vi "Get Incrementing Class Name.vi"() -> (3 "String":string)   [LabVIEW 2020, in "New Class Dialog.lvclass"]
uses:
  New Class Dialog.lvclass
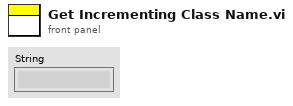
[diagram p1: front panel]
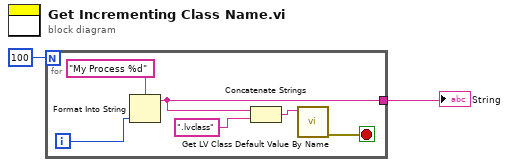
[diagram p0: block diagram]
diagram:
  n1 = for {
    N: 100 -> [_]
    tunnel: [w5] -> w2
    i -> [w7]
    stop <- w6 stop-if-true
    n2 = Format Into String(format string="My Process %d", w7) -> (resulting string=w5:string)  [unwired: 2 in, 1 out]
    n3 = Concatenate Strings(w5, ".lvclass" ("string")) -> (w4:string)
    n4 = call <vilib>:"Get LV Class Default Value By Name.vi"("class name"=w4) -> ("error out"=w6:errorcluster)  [unwired: 9 in, 1 out]
  }
  "String" <- w2
